vi "Setup AWG and Measure Resistance Only.vi"(4 "Settings":T2={"Level"=0.01, "Level Range"=0.1, "Limit"=1.0, "Limit Range"=6.0, "Sense"=1009} {"Sense" items=["Local"=1008, "Remote"=1009]}, 5 "cleanup script":string="BeamsOff", 6 "Published_ID":string="_Free", 7 "setup script":string="PullDown41v", 8 "error in (no error)":errorcluster, 9 "Pins":string[](array[string]), 10 "current level":dbl=0.01 format="%_6p", 11 "Semiconductor Module Context":T3) -> (0 "error out":errorcluster, 2 "R Array":dbl[](array[numeric]), 3 "Semiconductor Module Context Out":T3)   [LabVIEW 2013]
uses:
  <vilib>/NI_TestStand_SemiconductorModule/NI_TestStand_Semiconductor_Module.lvlibp/PinMap/General/SemiconductorModuleContext.ctl
  <instrlib>/niDCPower/nidcpower.llb/niDCPower Sense.ctl
  <instrlib>/niHSDIO/niHSDIO.llb/niHSDIO_ctl Trigger Script - trigID Values (Ring).ctl
  <instrlib>/niDCPower/nidcpower.llb/niDCPower Wait For Event - Event.ctl
  <vilib>/NI_TestStand_SemiconductorModule/NI_TestStand_Semiconductor_Module.lvlibp/PinMap/DC Power/PinToNIDCPowerSessions.vi
  <vilib>/NI_TestStand_SemiconductorModule/NI_TestStand_Semiconductor_Module.lvlibp/PinMap/General/Publish/PublishDataDoubleFunctionalTest.vi
  <vilib>/NI_TestStand_SemiconductorModule/NI_TestStand_Semiconductor_Module.lvlibp
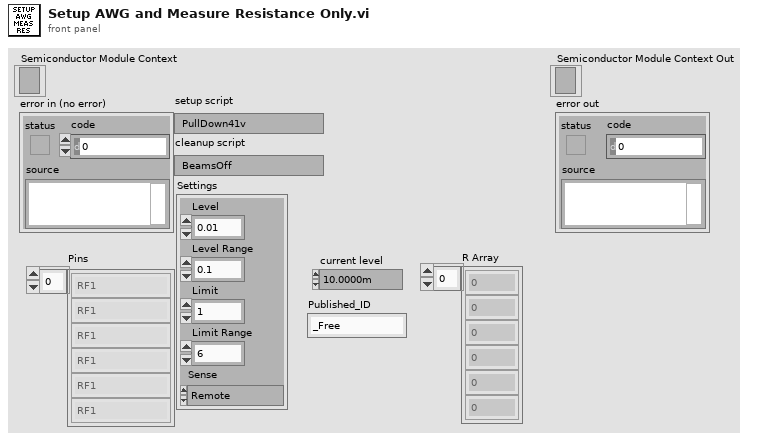
[diagram p1: front panel]
types:
  T1 = typedef "niDCPower Sense.ctl" = i32
  T2 = cluster{"Level":dbl, "Level Range":dbl, "Limit":dbl, "Limit Range":dbl, "Sense":T1}
  T3 = typedef "NI_TestStand_Semiconductor_Module.lvlibp/SemiconductorModuleContext.ctl" = refnum<k7>
  T4 = typedef "niHSDIO_ctl Trigger Script - trigID Values (Ring).ctl" = string
  T5 = typedef "niDCPower Wait For Event - Event.ctl" = i32
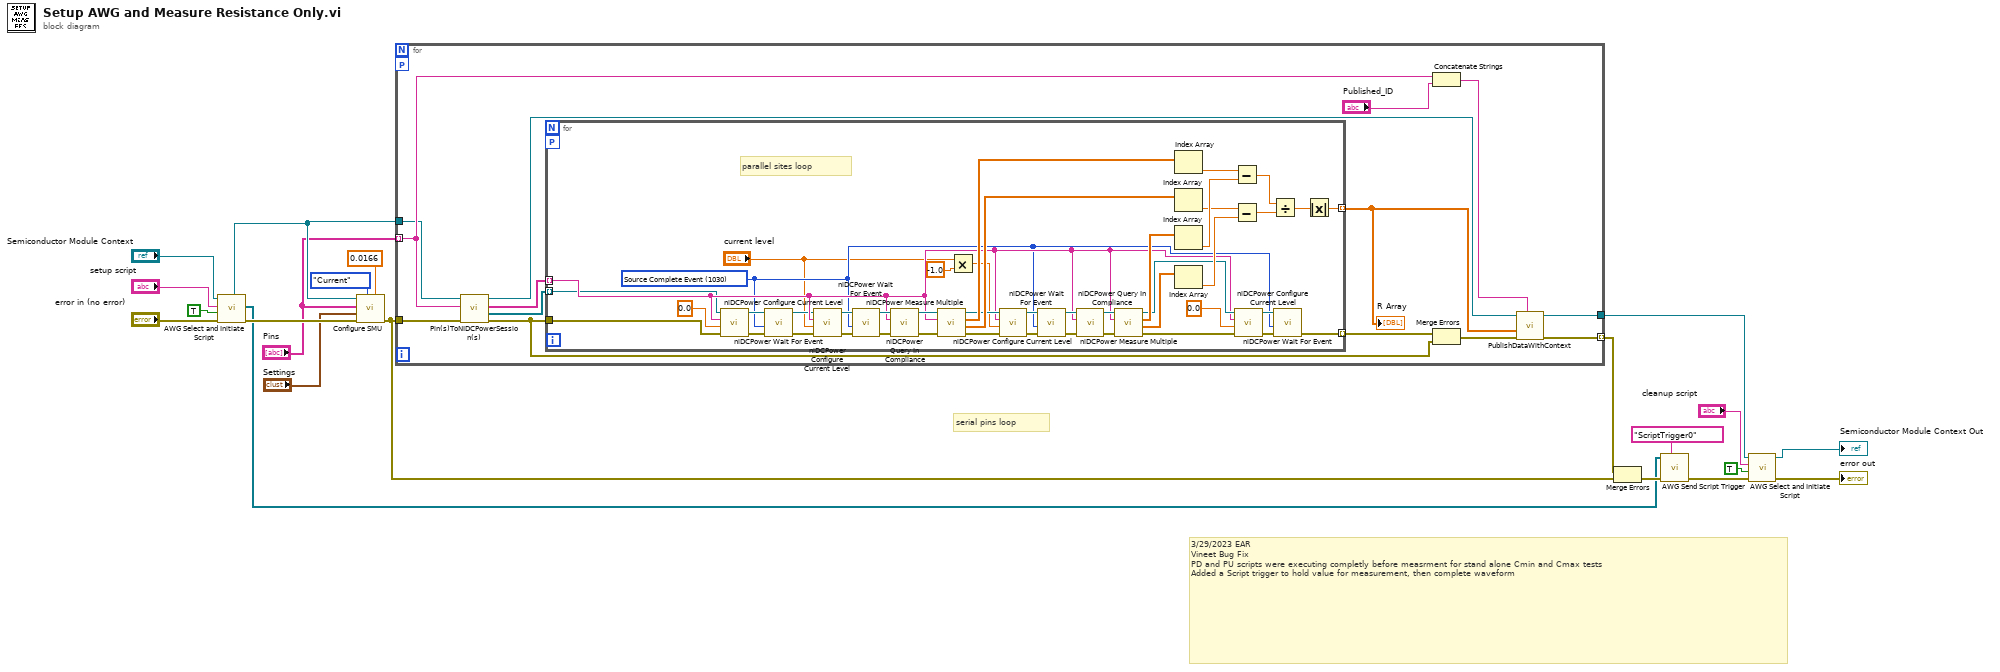
[diagram p0: block diagram]
diagram:
  # "3/29/2023 EAR\nVineet Bug Fix\nPD and PU scripts were executing completly before measrment for stand alone Cmin and Cmax tests\nAdded a Script trigger to hold value for measurement, then complete waveform"
  # "serial pins loop"
  n1 = call "AWG Select and Initiate Script.vi"("error in (no error)"="error in (no error)", "Wait for Completion"=TRUE, "script name"="setup script", "Semiconductor Module Context"="Semiconductor Module Context") -> ("error out"=w11:errorcluster, "Sessions Out"=w1:refnum<k15>[], "Semiconductor Module Context Out"=w9:T3)  [unwired: 5 in]
  n2 = call "Configure SMU.vi"("aperture time"=0.0166, "Source Mode"=enum16{"Voltage", "Current"}."Current", "error in (no error)"=w11, "Settings"="Settings", "Pins"="Pins", "Semiconductor Module Context"=w9) -> ("error out"=w10:errorcluster)  [unwired: 5 in]
  n3 = for {
    tunnel: [w30] -> w16
    tunnel: "Pins" -> [w27] mode=indexing
    tunnel: [w28] -> w21 mode=indexing
    workers-P: _ -> [_]
    tunnel: w10 -> [w23]
    tunnel: w9 -> [w22]
    n4 = call-poly <vilib>:"Pin(s)ToNIDCPowerSession(s).vi"("error in (no error)"=w23, "Pin"=w27, "Semiconductor Module Context"=w22) -> ("error out"=w32:errorcluster, "Instrument Sessions"=w34:refnum<k15>[], "Channel Lists"=w35:string[], "Semiconductor Module Context Out"=w31:T3)  [unwired: 4 in, 1 out]
    n5 = for {
      tunnel: w35 -> [w45] mode=indexing
      tunnel: w34 -> [w44] mode=indexing
      workers-P: _ -> [_]
      tunnel: w32 -> [w47]
      tunnel: [w78] -> w33 mode=indexing
      tunnel: [w67] -> w24 mode=indexing
      w40 = T5 1030 items=["Source Complete Event"=1030, "Measure Complete Event"=1031, "Sequence Iteration Complete Event"=1032, "Sequence Engine Done Event"=1033, "Pulse Complete Event"=1051, "Ready For Pulse Trigger Event"=1052] ("event")
      # "parallel sites loop"
      n6 = call <instrlib>:"niDCPower Configure Current Level.vi"("error in (no error)"=w47, "current level"=0.0, "channel name"=w45, "instrument handle"=w44) -> ("error out"=w48:errorcluster, "instrument handle out"=w43:refnum<k15>)  [unwired: 6 in]
      n7 = call <instrlib>:"niDCPower Wait For Event.vi"("error in (no error)"=w48, "event"=w40, "instrument handle"=w43) -> ("error out"=w46:errorcluster, "instrument handle out"=w42:refnum<k15>)  [unwired: 7 in]
      n8 = call <instrlib>:"niDCPower Configure Current Level.vi"("error in (no error)"=w46, "current level"="current level", "channel name"=w45, "instrument handle"=w42) -> ("error out"=w72:errorcluster, "instrument handle out"=w71:refnum<k15>)  [unwired: 6 in]
      n9 = call <instrlib>:"niDCPower Wait For Event.vi"("error in (no error)"=w72, "event"=w40, "instrument handle"=w71) -> ("error out"=w37:errorcluster, "instrument handle out"=w77:refnum<k15>)  [unwired: 7 in]
      n10 = call <instrlib>:"niDCPower Query In Compliance.vi"("error in (no error)"=w37, "channel name"=w45, "instrument handle"=w77) -> ("error out"=w73:errorcluster, "instrument handle out"=w74:refnum<k15>)  [unwired: 6 in, 1 out]
      n11 = call <instrlib>:"niDCPower Measure Multiple.vi"("error in (no error)"=w73, "channel name"=w45, "instrument handle"=w74) -> ("error out"=w52:errorcluster, "current measurements"=w68:dbl[], "voltage measurements"=w69:dbl[], "instrument handle out"=w50:refnum<k15>)  [unwired: 5 in]
      n12 = Multiply(x="current level", y=-1.0) -> (x*y=w39:dbl)
      n13 = call <instrlib>:"niDCPower Configure Current Level.vi"("error in (no error)"=w52, "current level"=w39, "channel name"=w45, "instrument handle"=w50) -> ("error out"=w62:errorcluster, "instrument handle out"=w61:refnum<k15>)  [unwired: 6 in]
      n14 = call <instrlib>:"niDCPower Wait For Event.vi"("error in (no error)"=w62, "event"=w40, "instrument handle"=w61) -> ("error out"=w36:errorcluster, "instrument handle out"=w65:refnum<k15>)  [unwired: 7 in]
      n15 = call <instrlib>:"niDCPower Query In Compliance.vi"("error in (no error)"=w36, "channel name"=w45, "instrument handle"=w65) -> ("error out"=w63:errorcluster, "instrument handle out"=w64:refnum<k15>)  [unwired: 6 in, 1 out]
      n16 = call <instrlib>:"niDCPower Measure Multiple.vi"("error in (no error)"=w63, "channel name"=w45, "instrument handle"=w64) -> ("error out"=w51:errorcluster, "current measurements"=w59:dbl[], "voltage measurements"=w60:dbl[], "instrument handle out"=w49:refnum<k15>)  [unwired: 5 in]
      n17 = Index Array(array=w69) -> (element=w56:dbl)  [unwired: 1 in]
      n18 = Index Array(array=w68) -> (element=w55:dbl)  [unwired: 1 in]
      n19 = Index Array(array=w60) -> (element=w58:dbl)  [unwired: 1 in]
      n20 = Index Array(array=w59) -> (element=w57:dbl)  [unwired: 1 in]
      n21 = Subtract(x=w56, y=w58) -> (x-y=w54:dbl)
      n22 = Subtract(x=w55, y=w57) -> (x-y=w53:dbl)
      n23 = call <instrlib>:"niDCPower Configure Current Level.vi"("error in (no error)"=w51, "current level"=0.0, "channel name"=w45, "instrument handle"=w49) -> ("error out"=w79:errorcluster, "instrument handle out"=w76:refnum<k15>)  [unwired: 6 in]
      n24 = Divide(x=w54, y=w53) -> (x/y=w70:dbl)
      n25 = call <instrlib>:"niDCPower Wait For Event.vi"("error in (no error)"=w79, "event"=w40, "instrument handle"=w76) -> ("error out"=w78:errorcluster)  [unwired: 7 in, 1 out]
      n26 = Absolute Value(x=w70) -> (abs(x)=w67:dbl)
    }
    "R Array" <- w24
    n27 = Concatenate Strings(w27, "Published_ID") -> (w25:string)
    n28 = Merge Errors(w33, w32) -> (w29:errorcluster)
    n29 = call-poly <vilib>:"PublishDataWithContext.vi"("Published Data Id"=w25, "error in (no error)"=w29, "Data In"=w24, "Semiconductor Module Context"=w31) -> ("error out"=w28:errorcluster, "Semiconductor Module Context Out"=w30:T3)  [unwired: 6 in]
  }
  n30 = Merge Errors(w21, w10) -> (w3:errorcluster)
  n31 = call "AWG Send Script Trigger.vi"("trigger id (script trigger 0)"=T4 "ScriptTrigger0", "error in (no error)"=w3, "AWG Sessions In"=w1) -> ("error out"=w2:errorcluster)  [unwired: 7 in, 1 out]
  n32 = call "AWG Select and Initiate Script.vi"("error in (no error)"=w2, "Wait for Completion"=TRUE, "script name"="cleanup script", "Semiconductor Module Context"=w16) -> ("error out"=→"error out":errorcluster, "Semiconductor Module Context Out"=→"Semiconductor Module Context Out":T3)  [unwired: 5 in, 1 out]
